vi "UI_GUI.vi"() -> ()   [LabVIEW 2014]
uses:
  <vilib>/addons/database/Connection.llb/DB Tools Open Connec (String).vi
  <vilib>/Utility/file.llb/Read From Spreadsheet File (string).vi
  Terminal-Global-SetValues.vi
  Terminal_Global_TestID.vi
  <vilib>/addons/database/_DB Variant To Data/Database Variant To Data.xnode
  <vilib>/addons/database/NI_Database_API.lvlib
panel:
  in  "取消":bool
  in  "选项卡控件":enum32{"选项卡 1", "选项卡 2", "选项卡 3", "选项卡 4"}(tab)
  in  "NEXT_1":bool caption="下一步"
  in  "试验人员姓名":string
  in  "试验名称":string
  out "试验日期":string
  out "布尔":bool
  in  "预载荷时间":dbl
  in  "径向液压缸加载压力":dbl
  in  "轴向液压缸加载压力":dbl
  in  "润滑油温度":dbl
  in  "轴承类型":enum32{"角接触球", "圆柱滚子"}(radio)
  in  "BACK_2":bool caption="上一步"
  in  "NEXT_2":bool caption="下一步"
  in  "供油流量":dbl
  in  "执行次数":dbl=1.0
  in  "下拉列表":u16(ring) items=["", "模板一", "模板二", "模板三"]
  in  "选择文件":path
  in  "BACK_3":bool caption="上一步"
  in  "NEXT_3":bool caption="下一步"
  in  "载荷谱表格":string[][](table)
  out "预载荷时间显示":dbl caption="预载荷时间"
  out "轴向加载压力显示":dbl caption="轴向液压缸加载压力"
  out "载荷谱表格显示":string[][](table) caption="载荷谱表格"
  out "润滑油温度显示":dbl caption="润滑油温度"
  out "轴承类型显示":string caption="轴承类型"
  in  "BACK_4":bool caption="上一步"
  out "试验日期显示":string caption="试验日期"
  out "试验人员姓名显示":string caption="试验人员姓名"
  out "试验名称显示":string caption="试验名称"
  out "径向加载压力显示":dbl caption="径向液压缸加载压力"
  out "供油流量显示":dbl caption="供油流量"
  in  "ok":bool
  # "轴承测试系统"
  # "试验信息输入"
  # "试验轴承类型"
  # "请选择"
  # "试验轴承润滑单元设定"
  # "L"
  # "℃"
  # "预载荷及高压顶起载荷设置"
  # "KN"
  # "KN"
  # "Min"
  # "载荷谱设置"
  # "选择载荷谱模板"
  # "导入载荷谱"
  # "请确认您输入的内容"
  # "试验轴承润滑单元参数"
  # "预载荷及高压顶起载荷设置"
  # "Min"
  # "KN"
  # "℃"
  # "KN"
  # "L"
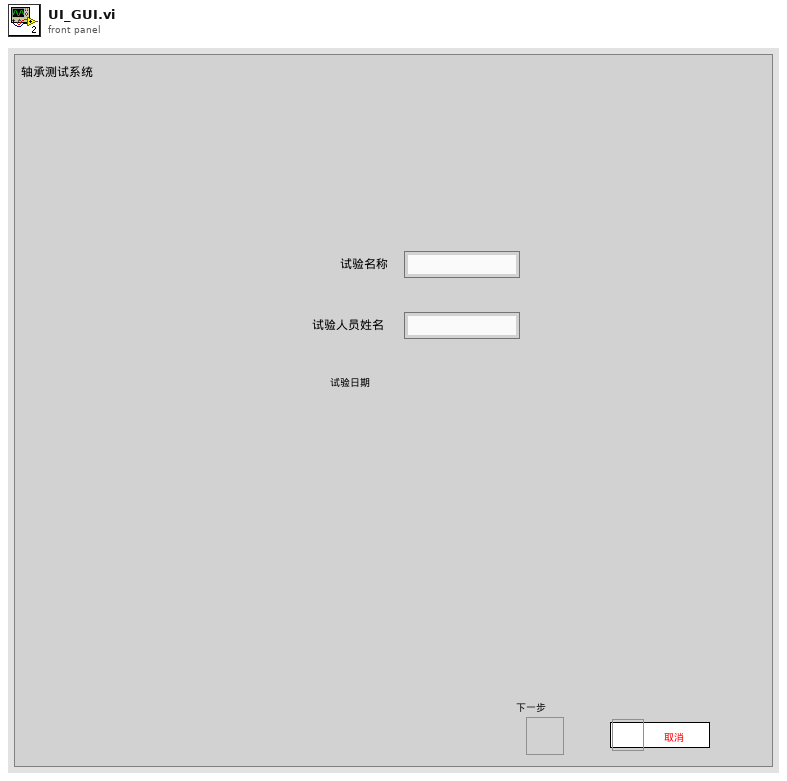
[diagram p1: front panel]
types:
  T1 = enum32{"选项卡 1", "选项卡 2", "选项卡 3", "选项卡 4", "选项卡 5", "选项卡 6", "选项卡 7"}
  T2 = typedef "LVStringsAndValuesArrayTypeDef_U16.ctl" = cluster{"String":string, "Value":u16}[]
  T3 = typedef "NI_Database_API.lvlib/Conn ObjectReference.ctl" = refnum<k1>
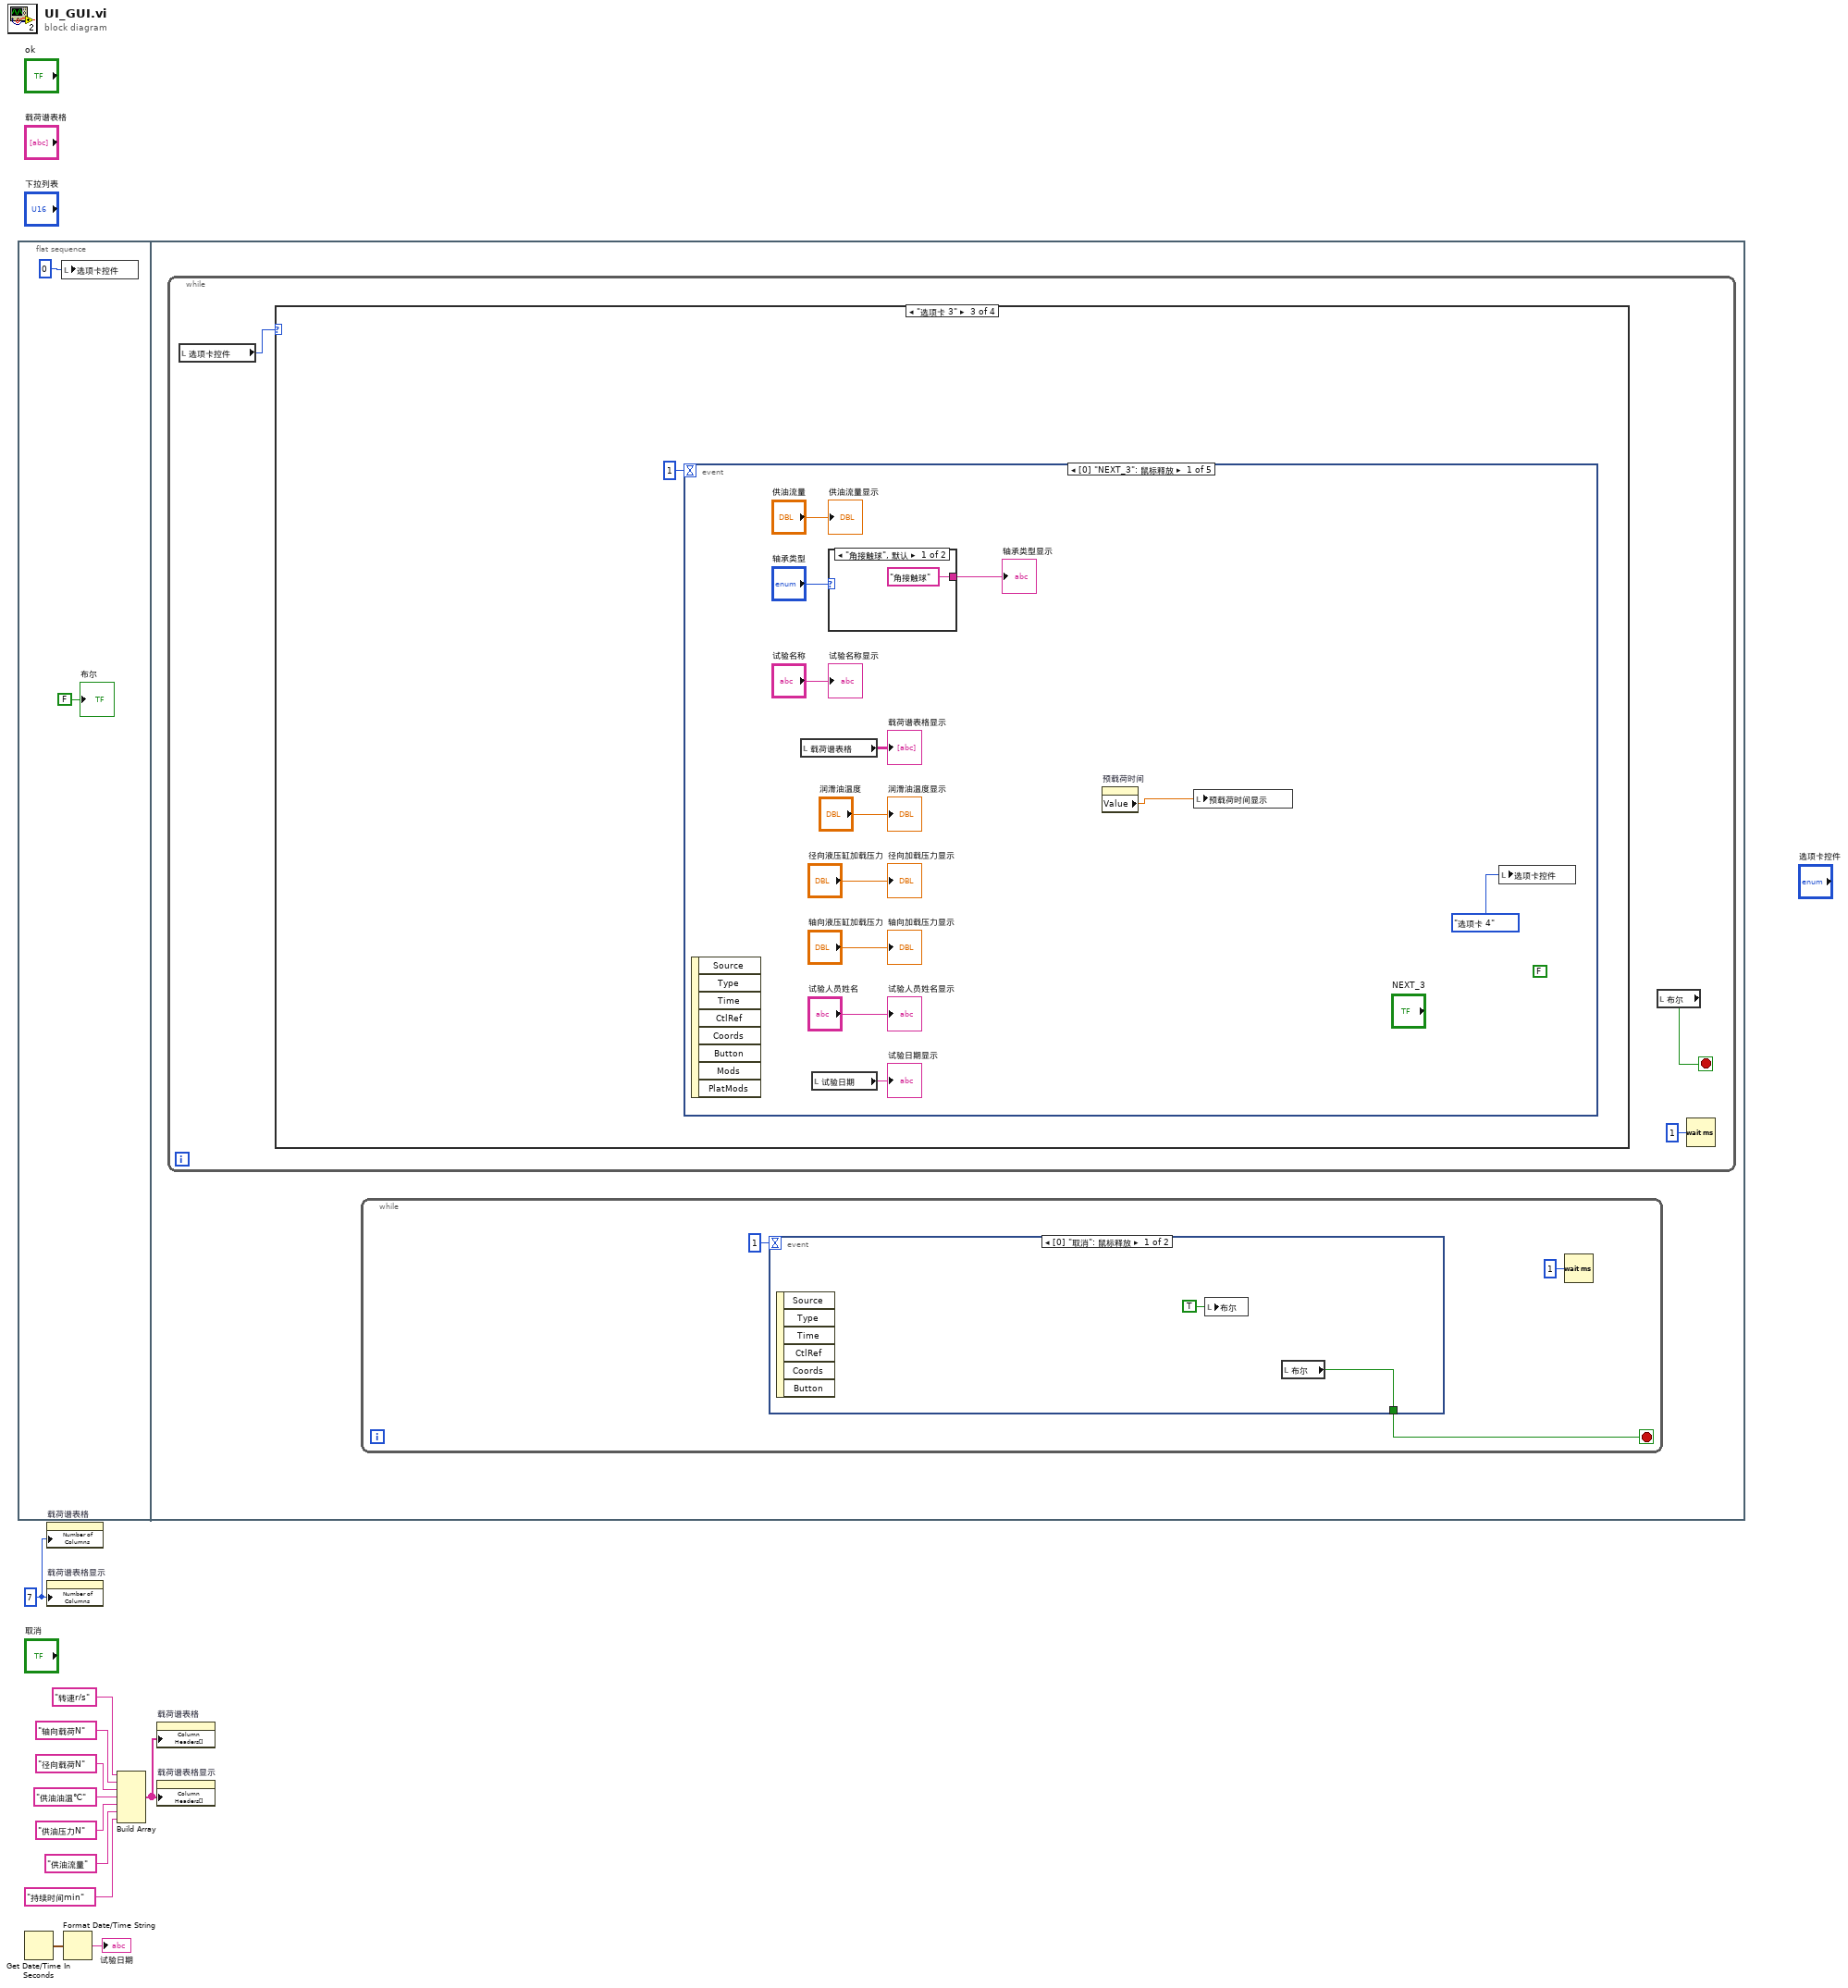
[diagram p0: block diagram]
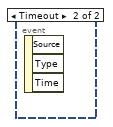
[diagram p2: hidden frame]
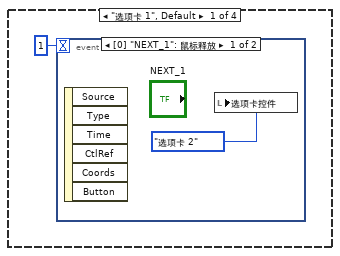
[diagram p3: hidden frame]
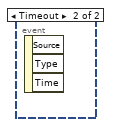
[diagram p4: hidden frame]
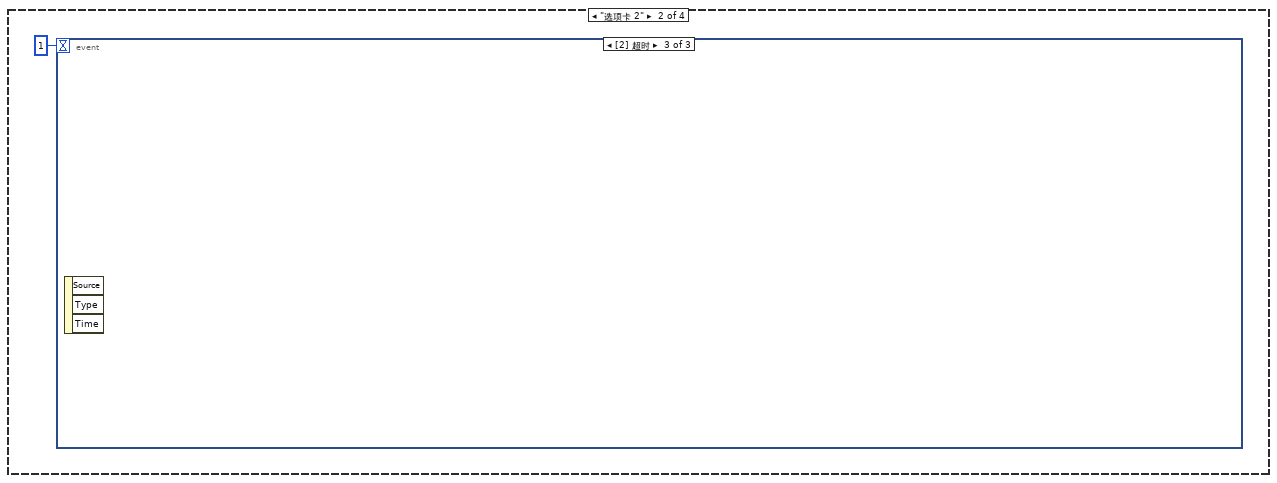
[diagram p5: hidden frame]
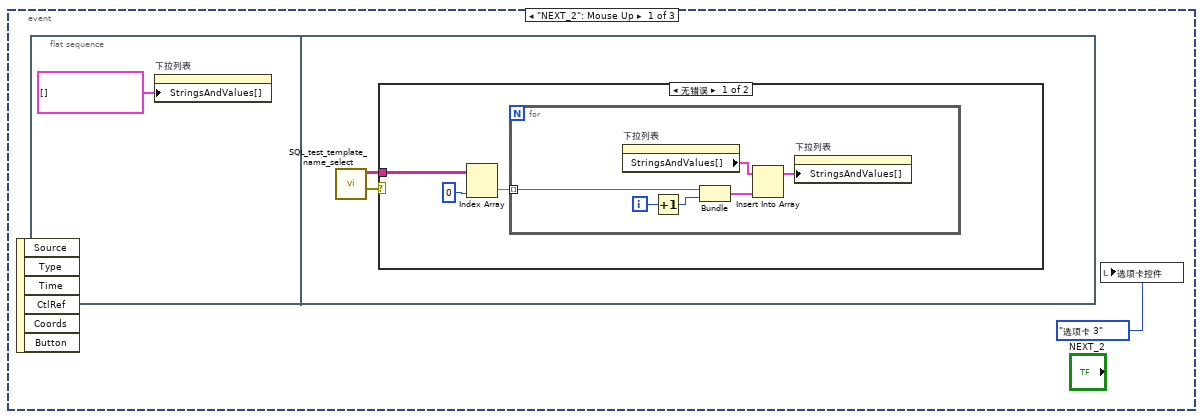
[diagram p6: hidden frame]
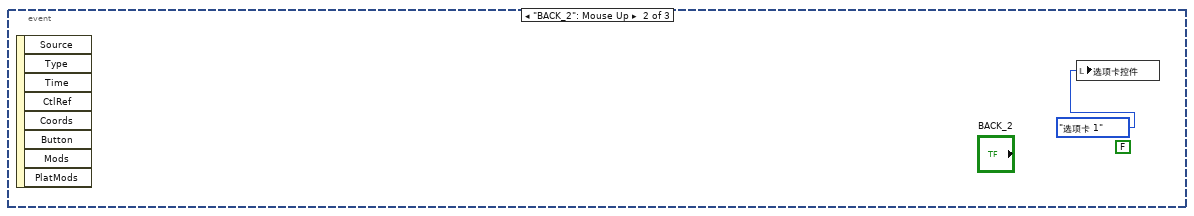
[diagram p8: hidden frame]
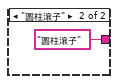
[diagram p9: hidden frame]
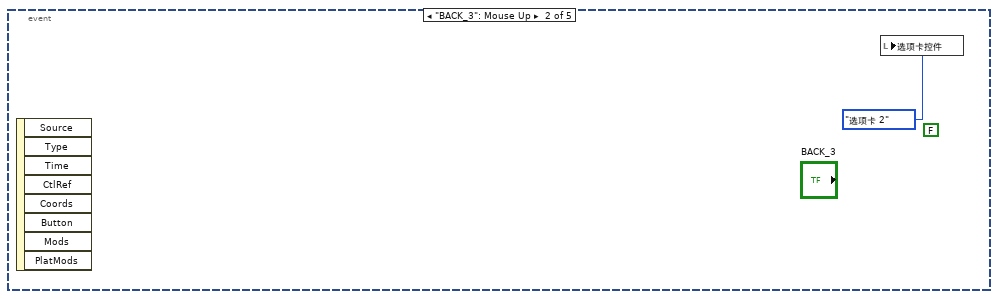
[diagram p10: hidden frame]
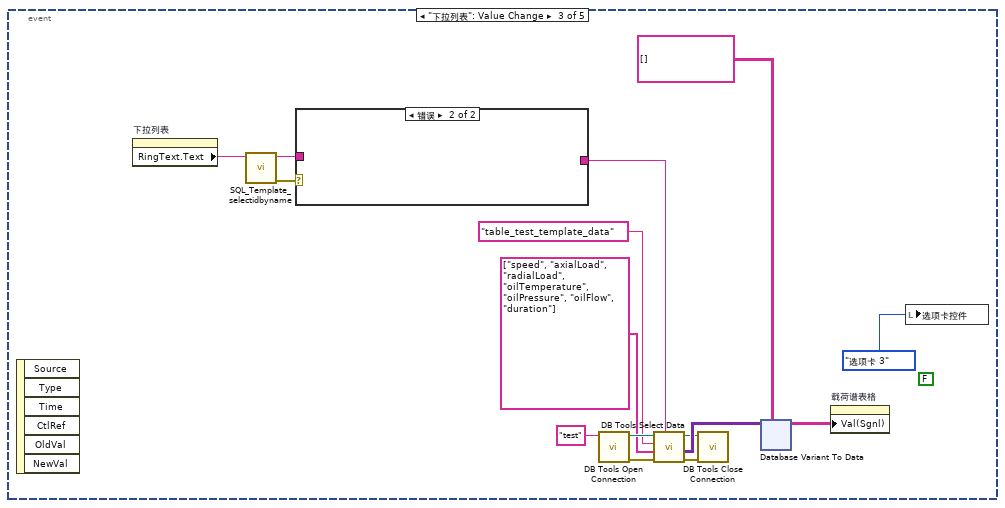
[diagram p11: hidden frame]
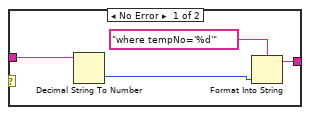
[diagram p12: hidden frame]
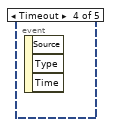
[diagram p13: hidden frame]
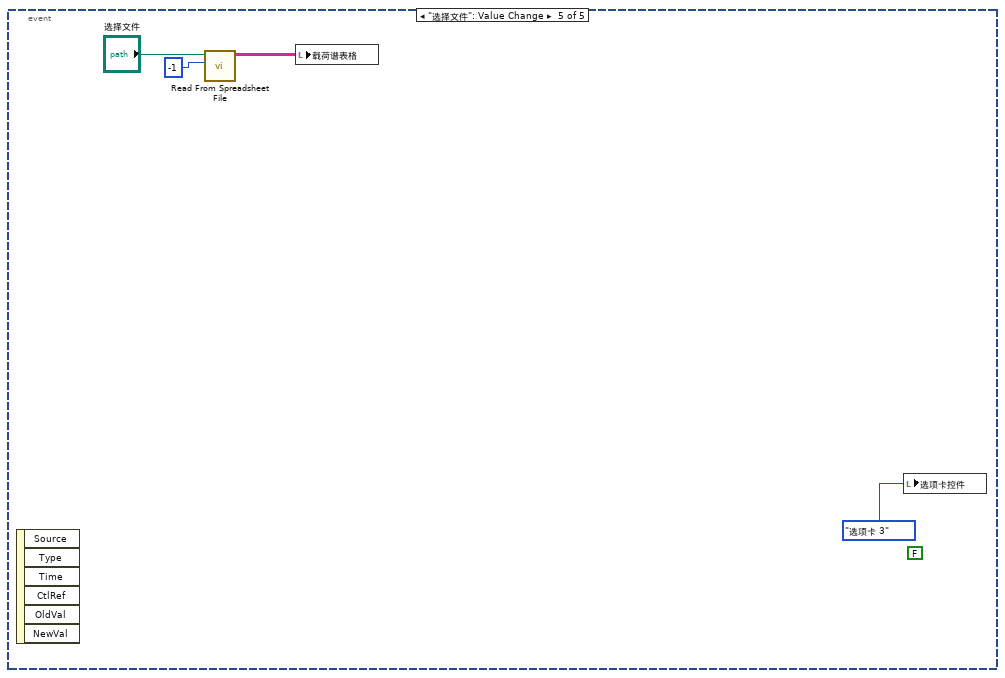
[diagram p14: hidden frame]
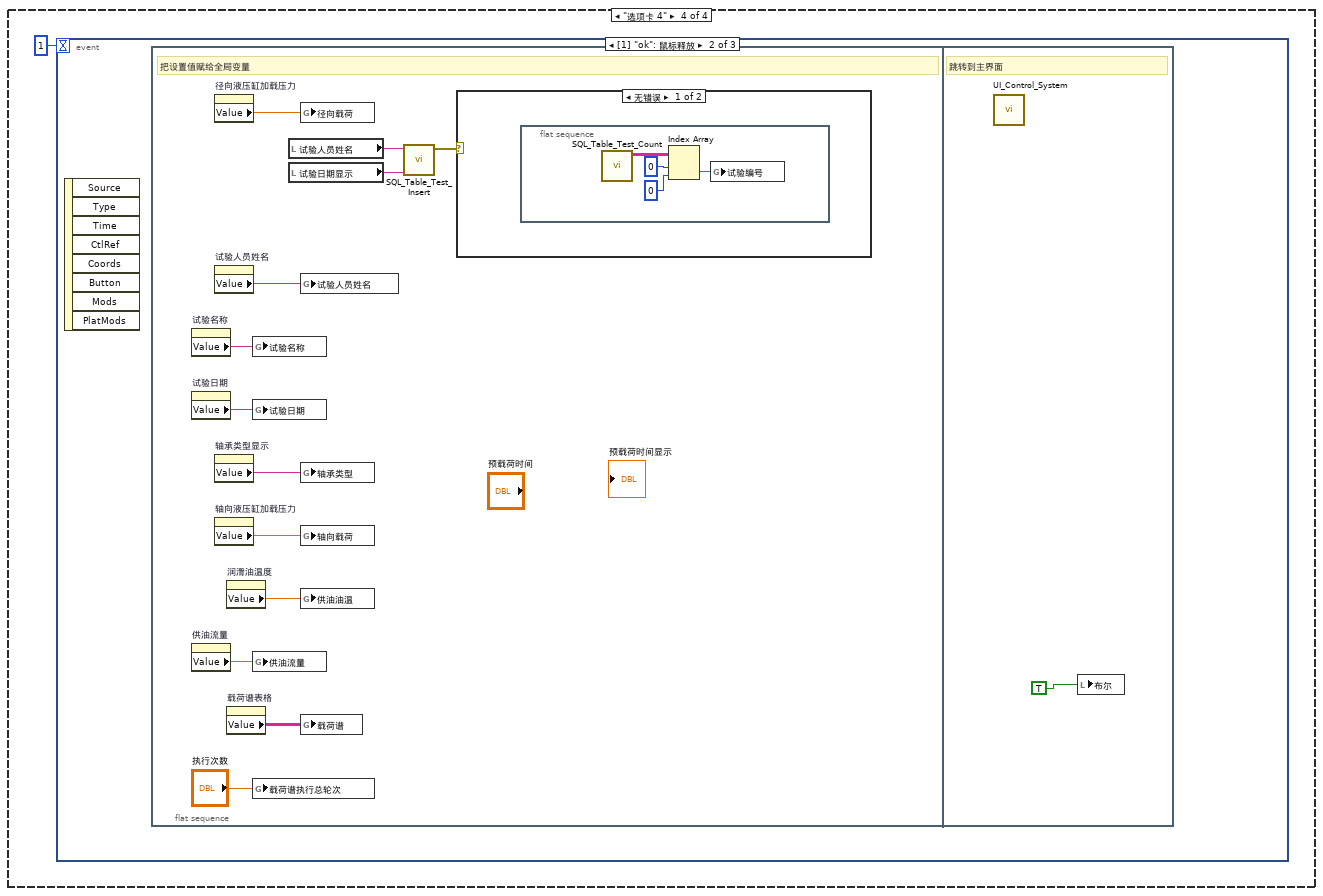
[diagram p15: hidden frame]
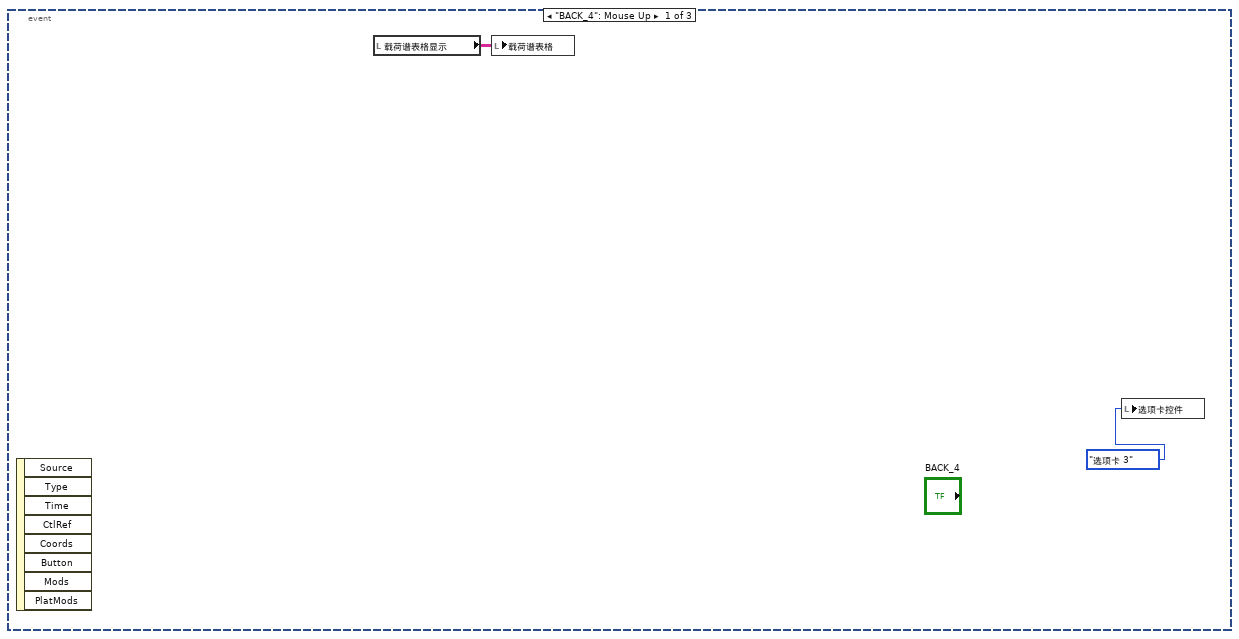
[diagram p16: hidden frame]
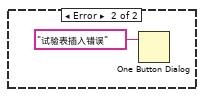
[diagram p17: hidden frame]
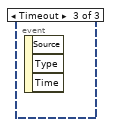
[diagram p18: hidden frame]
diagram:
  w1 = 7
  n1 = flat-sequence {
    frame #0 {
      n2 = local write "选项卡控件"(0) -> ()
      "布尔" <- FALSE ("布尔")
    }
    frame #1 {
      n3 = while {
        stop <- w19 stop-if-true
        n4 = local read "选项卡控件"() -> (w20:enum32{"选项卡 1", "选项卡 2", "选项卡 3", "选项卡 4"})
        n5 = case shown="\"选项卡 3\"" w20 {
          frame "选项卡 1", Default {
            n6 = event shown="[0] \"NEXT_1\": 鼠标释放" {
              selector: _ -> [_ _]
              dyn-events: _ -> [_ _]
              timeout: 1 -> [_ _]
              event "NEXT_1": Mouse Up {
                n7 = event-data() -> ()  [unwired: 1 in, 6 out]
                n8 = local write "选项卡控件"(T1."选项卡 2" ("选项卡控件")) -> ()
              }
              event Timeout {
                n9 = event-data() -> ()  [unwired: 1 in, 3 out]
              }
            }
          }
          frame "选项卡 2" {
            n10 = event shown="[2] 超时" {
              selector: _ -> [_ _ _]
              dyn-events: _ -> [_ _ _]
              timeout: 1 -> [_ _ _]
              event "NEXT_2": Mouse Up {
                n11 = event-data() -> ()  [unwired: 1 in, 6 out]
                n12 = flat-sequence {
                  frame #0 {
                    n13 = property on="下拉列表" class="Ring (严格)"("StringsAndValues[]"=cluster{string, dbl}[] []) -> ()  [unwired: 2 in, 2 out]
                  }
                  frame #1 {
                    n14 = call "SQL_test_template_name_select.vi"() -> ("error out"=w28:errorcluster, "模板名称"=w27:string[][])  [unwired: 10 in]
                    n15 = case shown="无错误" w28 {
                      tunnel: w27 -> [w31 _]
                      frame No Error {
                        n16 = Index Array(array=w31, index (col)=0 ("禁用的索引 (列)")) -> (element=w29:string[])  [unwired: 1 in]
                        n17 = for {
                          tunnel: w29 -> [w37] mode=indexing
                          i -> [w36]
                          n18 = property on="下拉列表" class="Ring (严格)"() -> ("StringsAndValues[]"=w34:T2)  [unwired: 2 in, 2 out]
                          n19 = Increment(x=w36) -> (x+1=w35:i32)
                          n20 = Bundle(w37, w35) -> (w33:cluster{string, i32})  [unwired: 1 in]
                          n21 = Insert Into Array(array=w34, new element=w33) -> (w32:T2)  [unwired: 1 in]
                          n22 = property on="下拉列表" class="Ring (严格)"("StringsAndValues[]"=w32) -> ()  [unwired: 2 in, 2 out]
                        }
                      }
                      frame Error {
                      }
                    }
                  }
                }
                n23 = local write "选项卡控件"(T1."选项卡 3" ("选项卡控件")) -> ()
              }
              event "BACK_2": Mouse Up {
                (unwired) FALSE
                n24 = event-data() -> ()  [unwired: 1 in, 8 out]
                n25 = local write "选项卡控件"(T1."选项卡 1" ("选项卡控件")) -> ()
              }
              event Timeout {
                n26 = event-data() -> ()  [unwired: 1 in, 3 out]
              }
            }
          }
          frame "选项卡 3" {
            n27 = event shown="[0] \"NEXT_3\": 鼠标释放" {
              selector: _ -> [_ _ _ _ _]
              dyn-events: _ -> [_ _ _ _ _]
              timeout: 1 -> [_ _ _ _ _]
              event "NEXT_3": Mouse Up {
                (unwired) FALSE
                n28 = event-data() -> ()  [unwired: 1 in, 8 out]
                n29 = local read "载荷谱表格"() -> (→"载荷谱表格显示":string[][])
                n30 = local read "试验日期"() -> (→"试验日期显示":string)
                n31 = case shown="\"角接触球\", 默认" "轴承类型" {
                  tunnel: ["角接触球" "圆柱滚子"] -> w43
                  frame "角接触球", Default {
                  }
                  frame "圆柱滚子" {
                  }
                }
                "轴承类型显示" <- w43
                n32 = property on="预载荷时间" class="DigNum (严格)"() -> ("Value"=w40:dbl)  [unwired: 2 in, 2 out]
                n33 = local write "预载荷时间显示"(w40) -> ()
                n34 = local write "选项卡控件"(enum32{"选项卡 1", "选项卡 2", "选项卡 3", "选项卡 4"}."选项卡 4" ("选项卡控件")) -> ()
                "试验名称显示" <- "试验名称"
                "试验人员姓名显示" <- "试验人员姓名"
                "供油流量显示" <- "供油流量"
                "径向加载压力显示" <- "径向液压缸加载压力"
                "轴向加载压力显示" <- "轴向液压缸加载压力"
                "润滑油温度显示" <- "润滑油温度"
              }
              event "BACK_3": Mouse Up {
                (unwired) FALSE
                n35 = event-data() -> ()  [unwired: 1 in, 8 out]
                n36 = local write "选项卡控件"(enum32{"选项卡 1", "选项卡 2", "选项卡 3", "选项卡 4"}."选项卡 2" ("选项卡控件")) -> ()
              }
              event "下拉列表": Value Change {
                (unwired) FALSE
                n37 = event-data() -> ()  [unwired: 1 in, 6 out]
                n38 = property on="下拉列表" class="Ring (严格)"() -> ("RingText.Text"=w58:string)  [unwired: 2 in, 2 out]
                n39 = call "SQL_Template_selectidbyname.vi"("模板名称"=w58) -> ("error out"=w57:errorcluster, "tempNo"=w56:string)  [unwired: 9 in]
                n40 = case shown="错误" w57 {
                  tunnel: [w70 _] -> w60
                  tunnel: w56 -> [w72 _]
                  frame No Error {
                    n41 = Decimal String To Number(string=w72) -> (number=w71:i32)  [unwired: 2 in, 1 out]
                    n42 = Format Into String(format string="where tempNo='%d'", w71) -> (resulting string=w70:string)  [unwired: 2 in, 1 out]
                  }
                  frame Error {
                  }
                }
                n43 = call-poly <vilib>:"DB Tools Open Connection.vi"("connection information"="test") -> ("error out"=w61:errorcluster, "connection reference"=w68:T3)  [unwired: 7 in]
                n44 = call <vilib>:"DB Tools Select Data.vi"("condition"=w60, "error in (no error)"=w61, "columns"=string[] ["speed", "axialLoad", "radialLoad", "oilTemperature", "oilPressure", "oilFlow", "duration"], "table"="table_test_template_data", "connection reference"=w68) -> ("error out"=w62:errorcluster, "data"=w65:variant[][], "connection reference out"=w63:T3)  [unwired: 1 in]
                n45 = call <vilib>:"DB Tools Close Connection.vi"("error in (no error)"=w62, "connection reference"=w63) -> ()  [unwired: 5 in, 1 out]
                n46 = xnode "Database Variant To Data"("database variant"=w65, "type"=string[][] []) -> ("data"=w59:string[][])  [unwired: 1 in, 1 out]
                n47 = property on="载荷谱表格" class="Tbl (严格)"("Val(Sgnl)"=w59) -> ()  [unwired: 2 in, 2 out]
                n48 = local write "选项卡控件"(T1."选项卡 3" ("选项卡控件")) -> ()
              }
              event Timeout {
                n49 = event-data() -> ()  [unwired: 1 in, 3 out]
              }
              event "选择文件": Value Change {
                (unwired) FALSE
                n50 = event-data() -> ()  [unwired: 1 in, 6 out]
                n51 = call-poly <vilib>:"Read From Spreadsheet File.vi"("number of rows (all:-1)"=-1, "file path (dialog if empty)"="选择文件") -> ("all rows"=w119:string[][])  [unwired: 5 in, 4 out]
                n52 = local write "载荷谱表格"(w119) -> ()
                n53 = local write "选项卡控件"(enum32{"选项卡 1", "选项卡 2", "选项卡 3", "选项卡 4"}."选项卡 3" ("选项卡控件")) -> ()
              }
            }
          }
          frame "选项卡 4" {
            n54 = event shown="[1] \"ok\": 鼠标释放" {
              selector: _ -> [_ _ _]
              dyn-events: _ -> [_ _ _]
              timeout: 1 -> [_ _ _]
              event "BACK_4": Mouse Up {
                n55 = event-data() -> ()  [unwired: 1 in, 8 out]
                n56 = local read "载荷谱表格显示"() -> (w124:string[][])
                n57 = local write "载荷谱表格"(w124) -> ()
                n58 = local write "选项卡控件"(enum32{"选项卡 1", "选项卡 2", "选项卡 3", "选项卡 4"}."选项卡 3" ("选项卡控件")) -> ()
              }
              event "ok": Mouse Up {
                n59 = event-data() -> ()  [unwired: 1 in, 8 out]
                n60 = flat-sequence {
                  frame #0 {
                    # "把设置值赋给全局变量"
                    n61 = property on="试验名称" class="Str"() -> ("Value"=w130:string)  [unwired: 2 in, 2 out]
                    n62 = property on="试验日期" class="Str"() -> ("Value"=w133:string)  [unwired: 2 in, 2 out]
                    n63 = property on="供油流量" class="DigNum (严格)"() -> ("Value"=w131:dbl)  [unwired: 2 in, 2 out]
                    n64 = property on="径向液压缸加载压力" class="DigNum (严格)"() -> ("Value"=w137:dbl)  [unwired: 2 in, 2 out]
                    n65 = property on="试验人员姓名" class="Str"() -> ("Value"=w134:string)  [unwired: 2 in, 2 out]
                    n66 = property on="轴承类型显示" class="Str"() -> ("Value"=w132:string)  [unwired: 2 in, 2 out]
                    n67 = property on="轴向液压缸加载压力" class="DigNum (严格)"() -> ("Value"=w136:dbl)  [unwired: 2 in, 2 out]
                    n68 = property on="润滑油温度" class="DigNum (严格)"() -> ("Value"=w135:dbl)  [unwired: 2 in, 2 out]
                    n69 = property on="载荷谱表格" class="Tbl (严格)"() -> ("Value"=w129:string[][])  [unwired: 2 in, 2 out]
                    n70 = global write "Terminal-Global-SetValues.vi" "试验名称"(w130) -> ()
                    n71 = global write "Terminal-Global-SetValues.vi" "试验日期"(w133) -> ()
                    n72 = global write "Terminal-Global-SetValues.vi" "供油流量"(w131) -> ()
                    n73 = global write "Terminal-Global-SetValues.vi" "载荷谱执行总轮次"("执行次数") -> ()
                    n74 = local read "试验人员姓名"() -> (w126:string)
                    n75 = local read "试验日期显示"() -> (w128:string)
                    n76 = global write "Terminal-Global-SetValues.vi" "径向载荷"(w137) -> ()
                    n77 = global write "Terminal-Global-SetValues.vi" "试验人员姓名"(w134) -> ()
                    n78 = global write "Terminal-Global-SetValues.vi" "轴承类型"(w132) -> ()
                    n79 = global write "Terminal-Global-SetValues.vi" "轴向载荷"(w136) -> ()
                    n80 = global write "Terminal-Global-SetValues.vi" "供油油温"(w135) -> ()
                    n81 = global write "Terminal-Global-SetValues.vi" "载荷谱"(w129) -> ()
                    n82 = call "SQL_Table_Test_Insert.vi"("试验开始日期"=w128, "用户名"=w126) -> ("error out"=w127:errorcluster)  [unwired: 9 in]
                    n83 = case shown="无错误" w127 {
                      frame No Error {
                        n84 = flat-sequence {
                          frame #0 {
                            n85 = call "SQL_Table_Test_Count.vi"() -> ("Data"=w141:string[][])  [unwired: 11 in]
                            n86 = Index Array(array=w141, index (row)=0 ("索引 (行)"), index (col)=0 ("禁用的索引 (列)")) -> (element=w138:string)
                            n87 = global write "Terminal_Global_TestID.vi" "试验编号"(w138) -> ()
                          }
                        }
                      }
                      frame Error {
                        n88 = One Button Dialog(message="试验表插入错误" ("消息")) -> ()  [unwired: 1 in, 1 out]
                      }
                    }
                  }
                  frame #1 {
                    # "跳转到主界面"
                    n89 = call "UI_Control_System.vi"() -> ()  [unwired: 12 in]
                    n90 = local write "布尔"(TRUE) -> ()
                  }
                }
              }
              event Timeout {
                n91 = event-data() -> ()  [unwired: 1 in, 3 out]
              }
            }
          }
        }
        n92 = local read "布尔"() -> (w19:bool)
        n93 = Wait (ms)(milliseconds to wait=u32 1 ("等待时间（毫秒）")) -> ()  [unwired: 1 out]
      }
      n94 = while {
        stop <- w16 stop-if-true
        n95 = event shown="[0] \"取消\": 鼠标释放" {
          selector: _ -> [_ _]
          dyn-events: _ -> [_ _]
          timeout: 1 -> [_ _]
          tunnel: [w17 _] -> w16
          event "取消": Mouse Up {
            n96 = event-data() -> ()  [unwired: 1 in, 6 out]
            n97 = local write "布尔"(TRUE ("布尔")) -> ()
            n98 = local read "布尔"() -> (w17:bool)
          }
          event Timeout {
            n99 = event-data() -> ()  [unwired: 1 in, 3 out]
          }
        }
        n100 = Wait (ms)(milliseconds to wait=u32 1 ("等待时间（毫秒）")) -> ()  [unwired: 1 out]
      }
    }
  }
  n101 = Get Date/Time In Seconds() -> (seconds since 1Jan1904=w4:timestamp)
  n102 = property on="载荷谱表格" class="Tbl (严格)"("Number of Columns"=w1) -> ()  [unwired: 2 in, 2 out]
  n103 = property on="载荷谱表格显示" class="Tbl (严格)"("Number of Columns"=w1) -> ()  [unwired: 2 in, 2 out]
  n104 = Format Date/Time String(seconds (now)=w4) -> (date/time string=→"试验日期":string)  [unwired: 2 in]
  n105 = Build Array("转速r/s", "轴向载荷N", "径向载荷N", "供油油温℃", "供油压力N", "供油流量", "持续时间min") -> (w2:string[])
  n106 = property on="载荷谱表格" class="Tbl (严格)"("Column Headers[]"=w2) -> ()  [unwired: 2 in, 2 out]
  n107 = property on="载荷谱表格显示" class="Tbl (严格)"("Column Headers[]"=w2) -> ()  [unwired: 2 in, 2 out]
